vi "ConvertBetweenXYandPixel.vi"(8 "XYtoPixels":bool=TRUE, 9 "PointToConvert":cluster{sgl, sgl}, 10 "HomeXY(pixels)":cluster{dbl, dbl}, 11 "Pixel/mm":dbl format="%#_13g") -> (3 "Point":cluster{sgl, sgl})   [LabVIEW 2017]
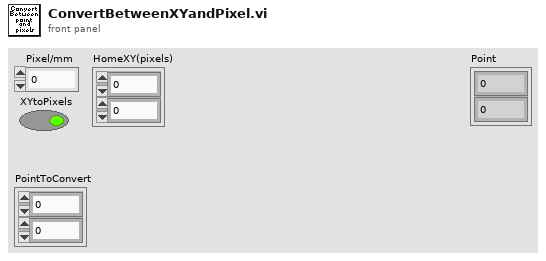
[diagram p1: front panel]
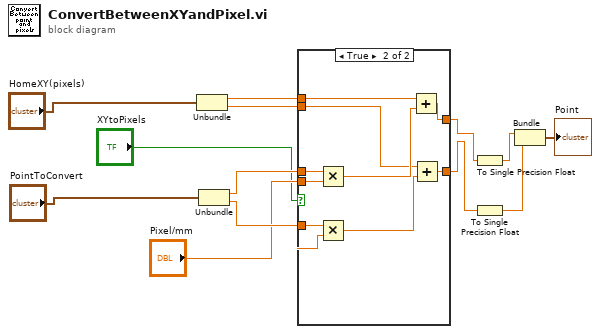
[diagram p0: block diagram]
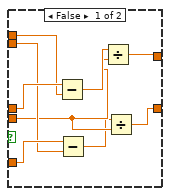
[diagram p2: hidden frame]
diagram:
  n1 = Unbundle("HomeXY(pixels)") -> (w8:dbl, w7:dbl)
  n2 = Unbundle("PointToConvert") -> (w11:sgl, w10:sgl)
  n3 = case shown="True" "XYtoPixels" {
    tunnel: w11 -> [w22 w31]
    tunnel: w10 -> [w20 w30]
    tunnel: "Pixel/mm" -> [w17 w29]
    tunnel: w8 -> [w21 w28]
    tunnel: w7 -> [w19 w26]
    tunnel: [w15 w24] -> w4
    tunnel: [w14 w23] -> w3
    frame False {
      n4 = Subtract(x=w22, y=w21) -> (x-y=w18:dbl)
      n5 = Subtract(x=w20, y=w19) -> (x-y=w16:dbl)
      n6 = Divide(x=w18, y=w17) -> (x/y=w15:dbl)
      n7 = Divide(x=w16, y=w17) -> (x/y=w14:dbl)
    }
    frame True {
      n8 = Multiply(x=w31, y=w29) -> (x*y=w27:dbl)
      n9 = Multiply(x=w30, y=w29) -> (x*y=w25:dbl)
      n10 = Add(x=w28, y=w27) -> (x+y=w24:dbl)
      n11 = Add(x=w26, y=w25) -> (x+y=w23:dbl)
    }
  }
  n12 = To Single Precision Float(number=w4) -> (single precision float=w2:sgl)
  n13 = To Single Precision Float(number=w3) -> (single precision float=w1:sgl)
  n14 = Bundle(w2, w1) -> (→"Point":cluster{sgl, sgl})  [unwired: 1 in]
